vi "PID Controller.vi"(1 "Auto?":bool=TRUE, 2 "u_man [V]":dbl, 7 "Process Variable":dbl format="%.2f", 11 "PID Parameters":cluster{"Kp":dbl, "Ti [s]":dbl, "Td [s]":dbl}={"Kp"=1.0, "Ti [s]"=5.0, "Td [s]"=0.0}, 13 "Setpoint [20-50deg]":dbl=30.0) -> (8 "u":dbl format="%.2f")   [LabVIEW 2018]
uses:
  <vilib>/addons/control/pid/pid.llb/PID Advanced (DBL).vi
  <vilib>/addons/control/pid/NI_PID_pid.lvlib
panel:
  # "This is the built-in PID controller in LabVIEW"
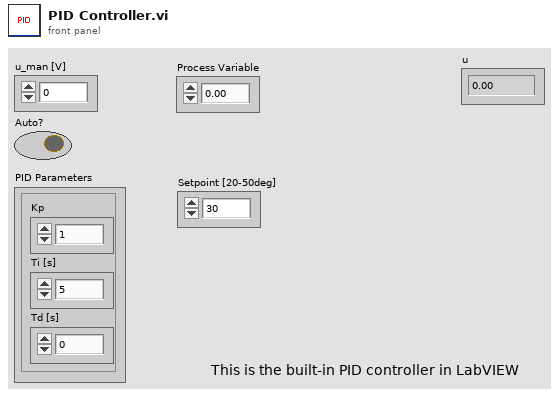
[diagram p1: front panel]
types:
  T1 = cluster{"Kc Scaling":i32, "Ti Scaling":i32, "Td Scaling":i32}
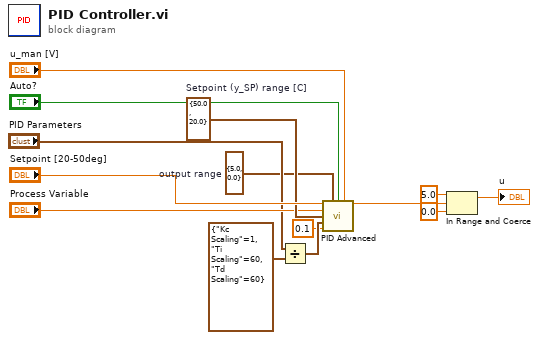
[diagram p0: block diagram]
diagram:
  w2 = cluster{"output high":dbl, "output low":dbl} {"output high"=5.0, "output low"=0.0}  # output range
  w9 = cluster{"Setpoint high":dbl, "Setpoint low":dbl} {"Setpoint high"=50.0, "Setpoint low"=20.0}  # Setpoint (y_SP) range [C]
  n1 = Divide(x="PID Parameters", y=T1 {"Kc Scaling"=1, "Ti Scaling"=60, "Td Scaling"=60} ("PID Param Scaling")) -> (x/y=w10:cluster{dbl, dbl, dbl})
  n2 = call-poly <vilib>:"PID Advanced.vi"("setpoint"="Setpoint [20-50deg]", "output range"=w2, "auto? (T)"="Auto?", "manual control"="u_man [V]", "process variable"="Process Variable", "setpoint range"=w9, "PID gains"=w10, "dt (s)"=0.1) -> ("output"=w5:dbl)  [unwired: 6 in, 1 out]
  n3 = In Range and Coerce(upper limit=5.0, x=w5, lower limit=0.0) -> (coerced(x)=→"u":dbl)  [unwired: 1 out]
